vi "Main.vi"() -> ()   [LabVIEW 2018]
doc: "This Continuous Measurement sample project is based on the Queued Message Handler template.\n\nThe Event Handling Loop generates messages based on user interface actions.\n\nThe Message Handling Loop processes messages generated by the Event Handling Loop, or by other messages. There are also Acquisition and Logging message handling loop subVIs, and a chart updating loop."
uses:
  controls/UI Data.ctl
  controls/UI State.ctl
  support/Message Queue/Enqueue Message (Single).vi
  GlobalVariable/GlobalLongueurOnde.vi
  GlobalVariable/GlobalSet0.vi
  GlobalVariable/GlobalDefaultFolderPath.vi
  <vilib>/Utility/error.llb/Error Cluster From Error Code.vi
  <vilib>/ErrorRing/Error Ring.xnode
  Acquisition/Acquisition.lvlib
  support/User Event - Stop/User Event - Stop.lvlib
  support/Message Queue/Message Queue.lvlib
panel:
  out "Pos Y":dbl
  out "Pos X":dbl
  out "?":dbl[][](graph)
  in  "Mise à 0":bool
  in  "Longueur d'onde du laser":dbl
  in  "Exit":bool
  out "Data":waveform(dbl)[](graph)
  out "Array":variant[](array[variant])
  out "Status":string
  out "Puissance Instantannée":dbl
  in  "Start":bool
  in  "Stop":bool
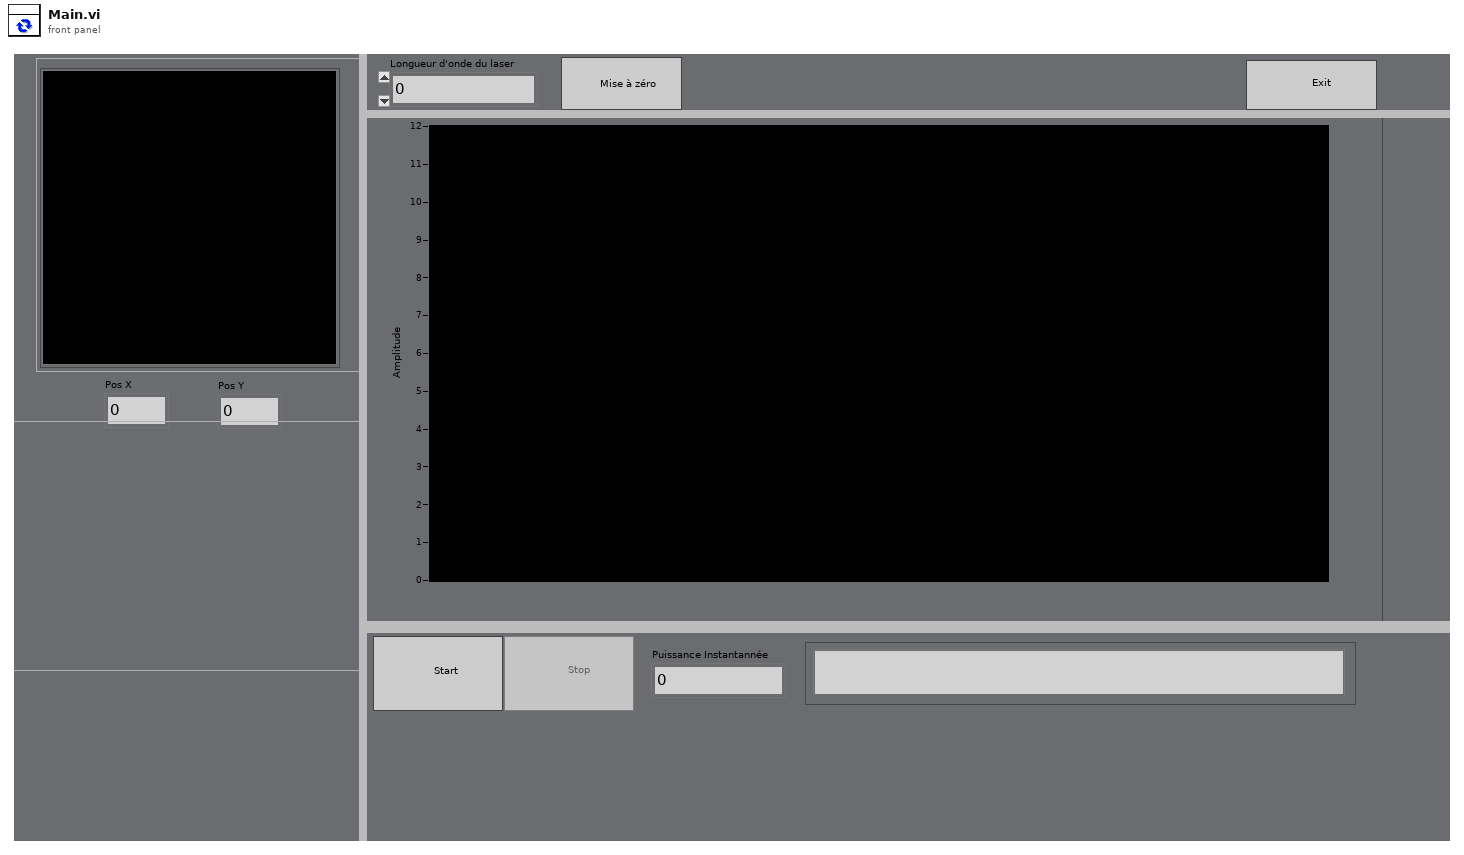
[diagram p1: front panel]
types:
  T1 = typedef "UI State.ctl" = enum16{"Idle", "Acquiring and Logging", "Waiting for Exit", "Waiting for Exit (Acq Stopped)", "Waiting for Exit (Log Stopped)", "Waiting for Stop", "Waiting for Stop (Acq Stopped)", "Waiting for Stop (Log Stopped)"}
  T2 = typedef "UI Data.ctl" = cluster{"Start Ref":refnum<vi>, "Stop Ref":refnum<vi>, "Settings Ref":refnum<vi>, "Exit Ref":refnum<vi>, "Status Ref":refnum<vi>, "Data Ref":refnum<vi>, "Longueur d'onde du laser":refnum<vi>, "Set 0 Ref":refnum<vi>}
  T3 = cluster{"UI":refnum<queue>, "Acquisition":refnum<queue>}
  T4 = enum16{"open", "replace", "create", "open or create", "replace or create", "replace or create with confirmation"}
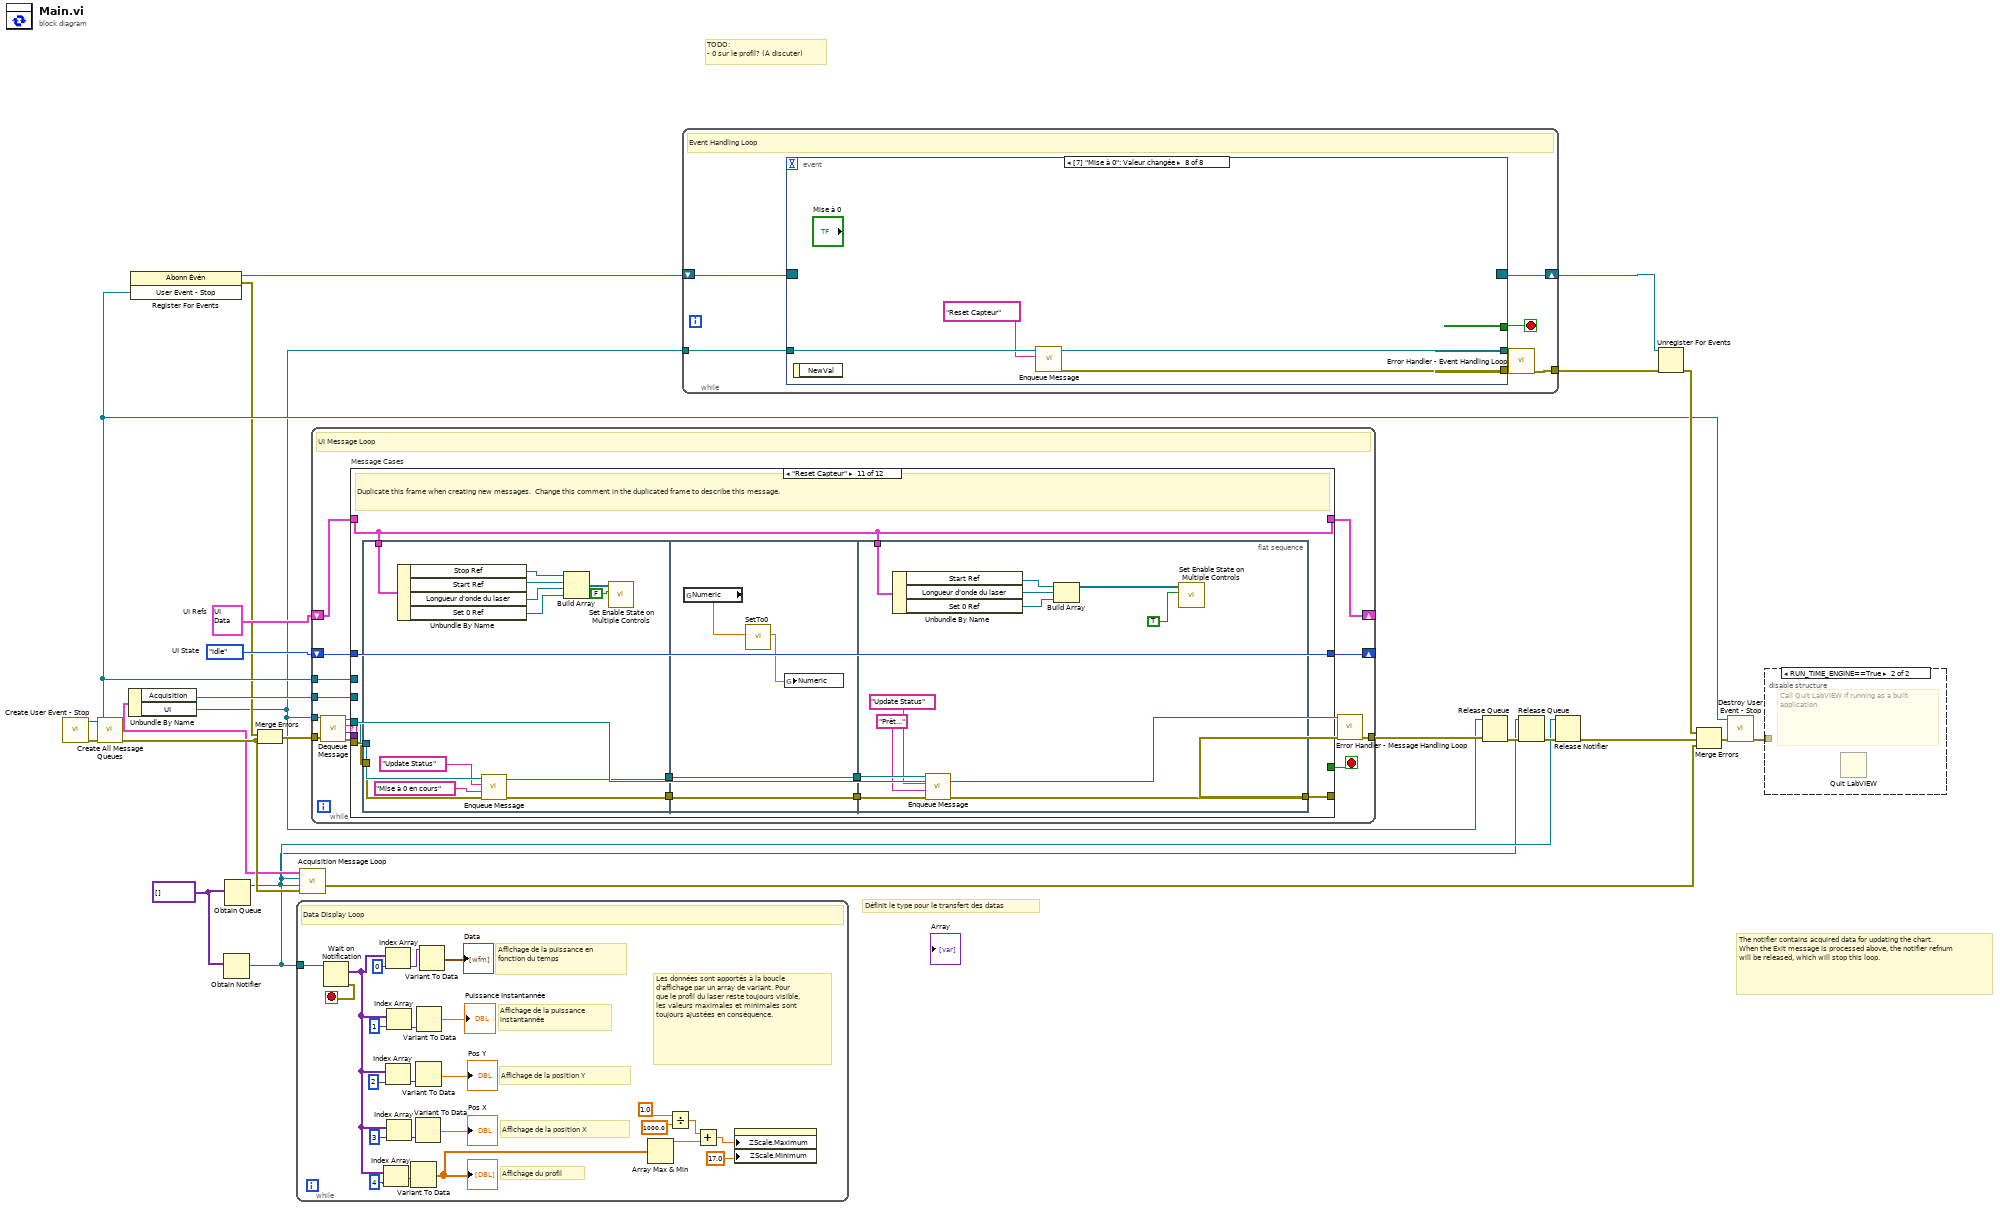
[diagram p0: block diagram]
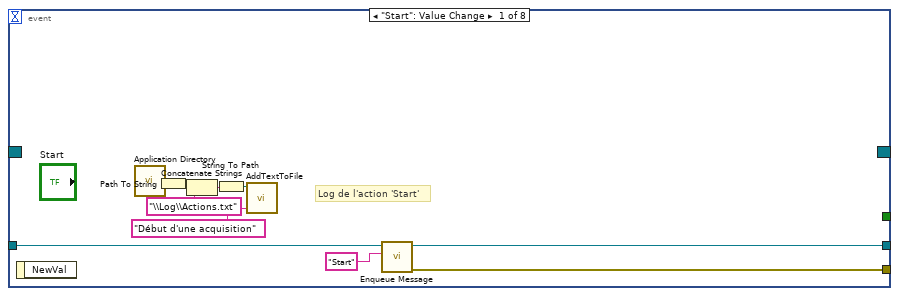
[diagram p3: hidden frame]
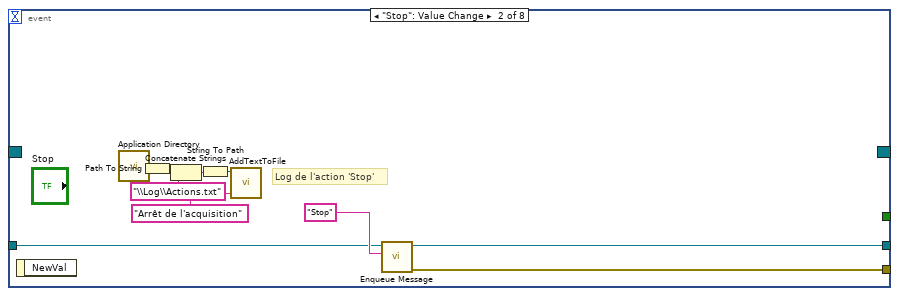
[diagram p4: hidden frame]
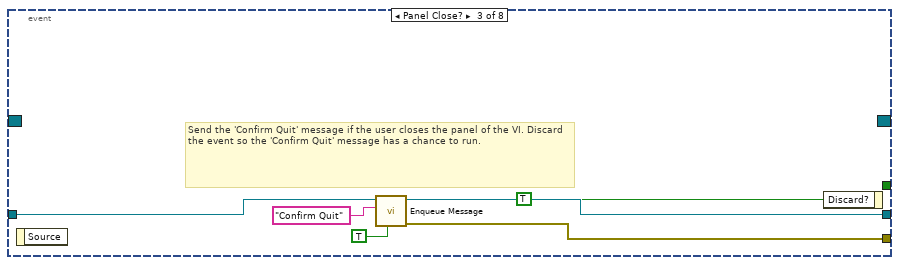
[diagram p5: hidden frame]
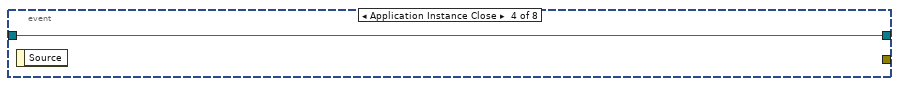
[diagram p6: hidden frame]
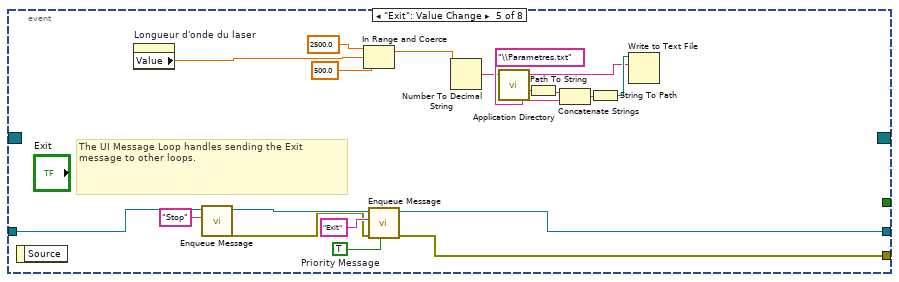
[diagram p7: hidden frame]
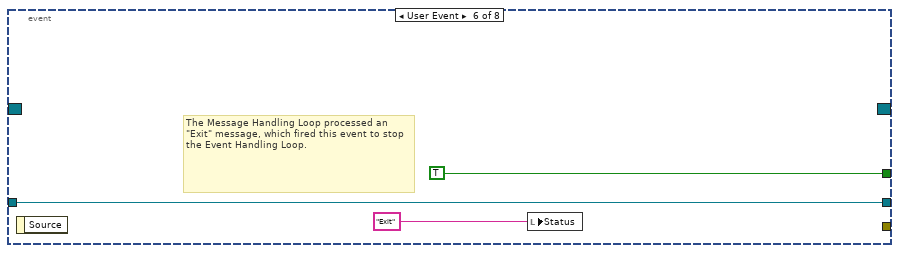
[diagram p8: hidden frame]
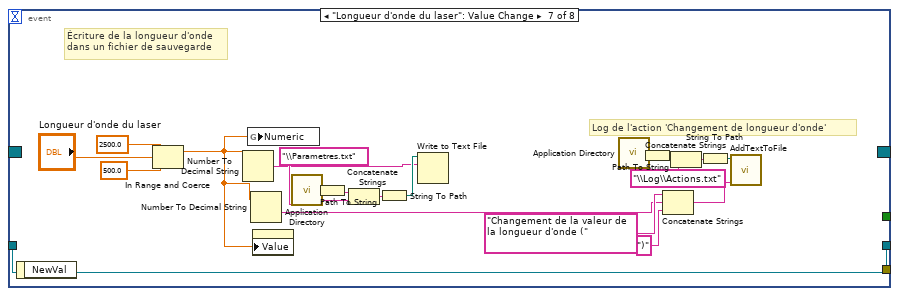
[diagram p9: hidden frame]
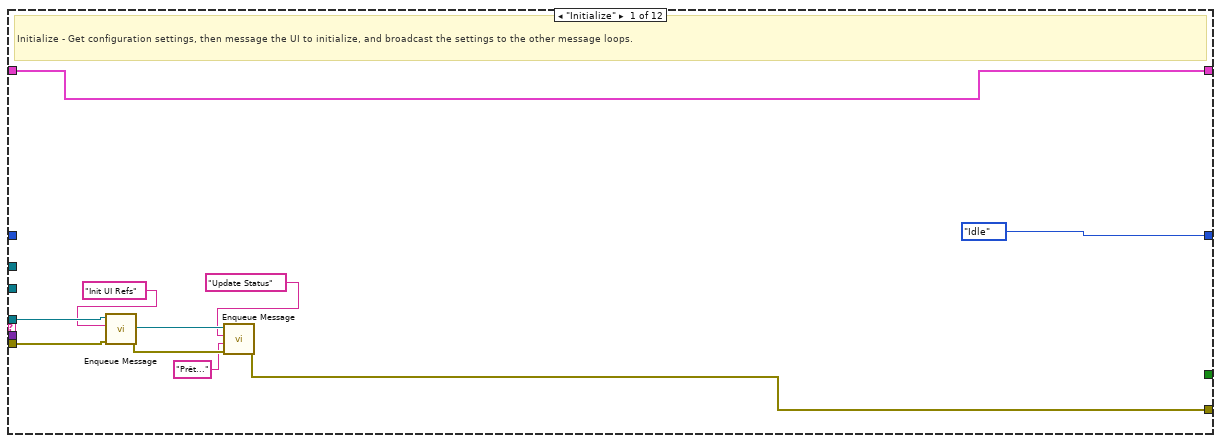
[diagram p10: hidden frame]
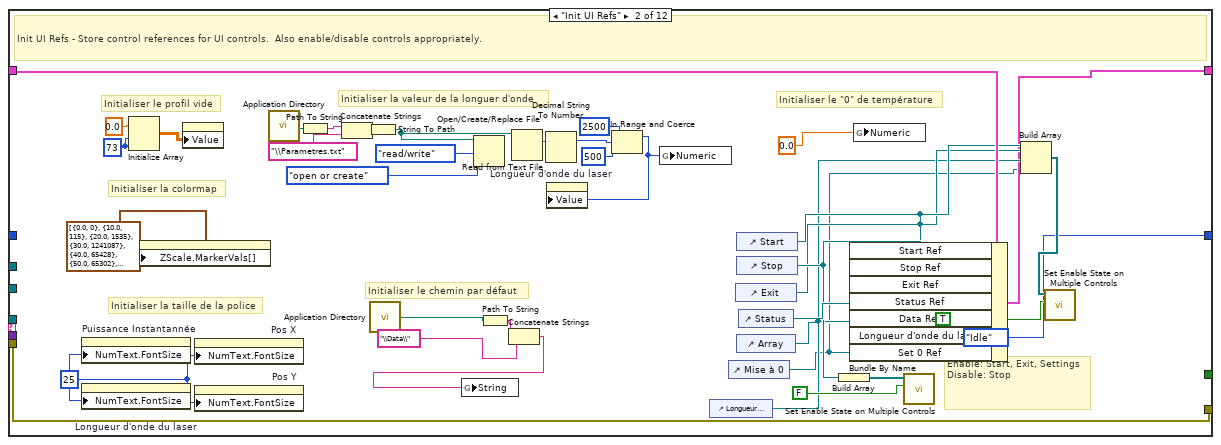
[diagram p11: hidden frame]
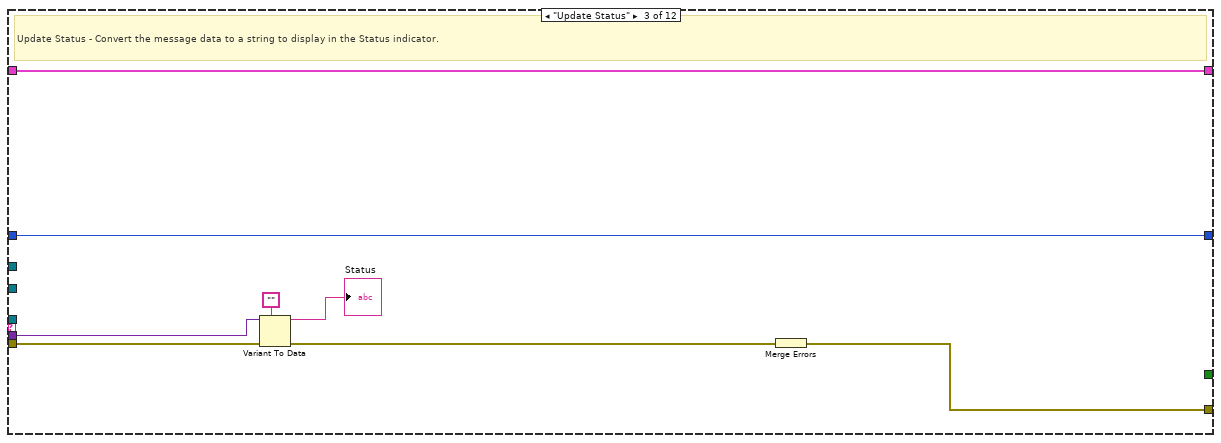
[diagram p12: hidden frame]
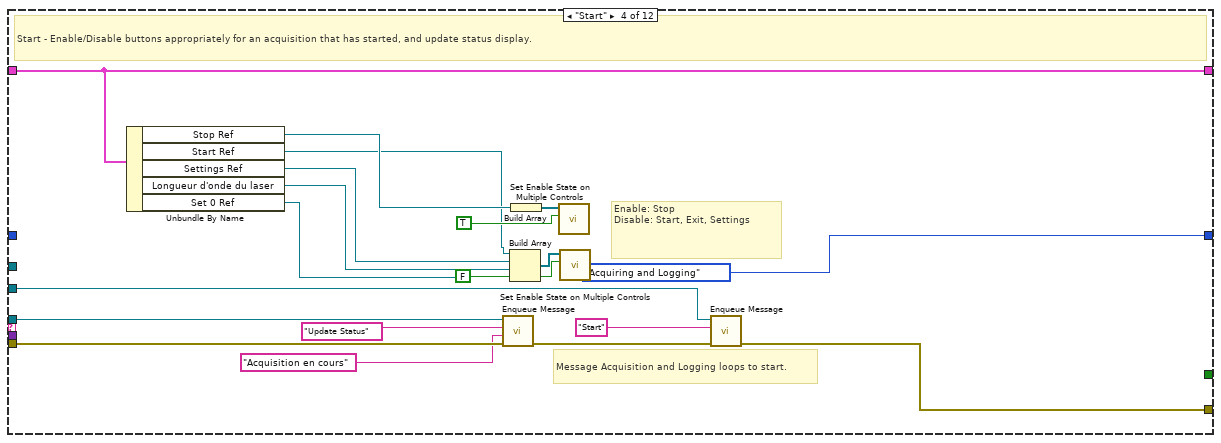
[diagram p13: hidden frame]
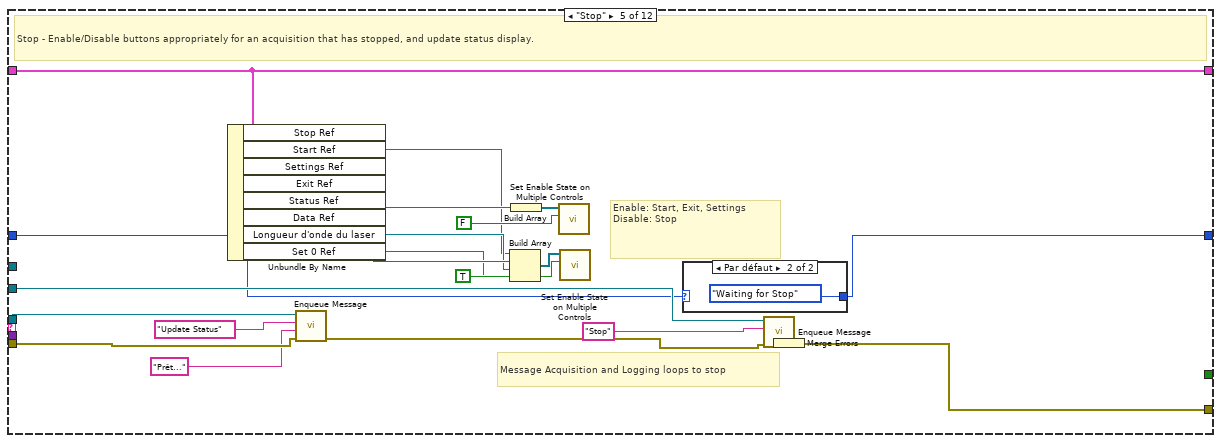
[diagram p14: hidden frame]
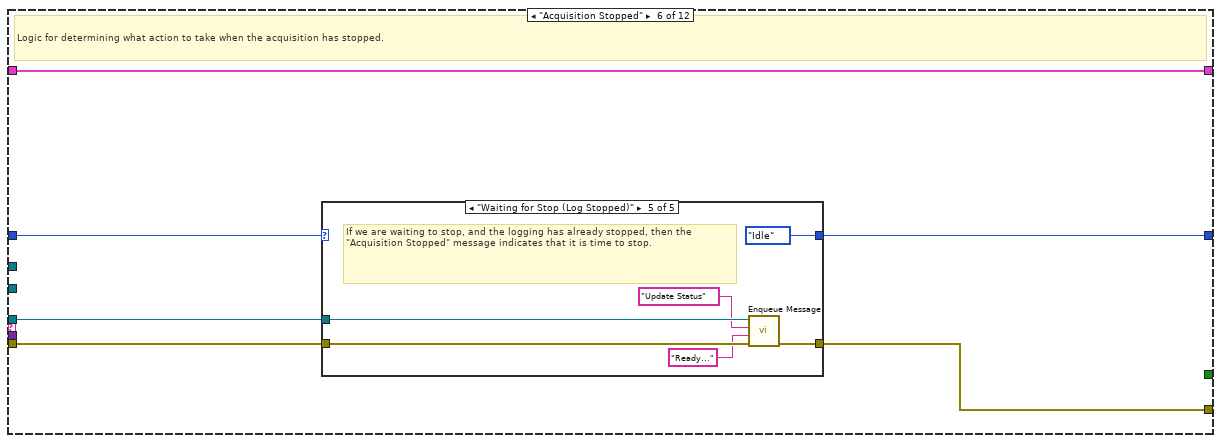
[diagram p16: hidden frame]
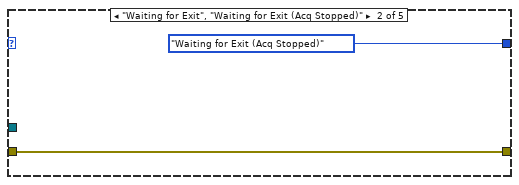
[diagram p18: hidden frame]
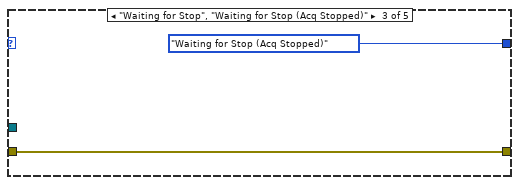
[diagram p19: hidden frame]
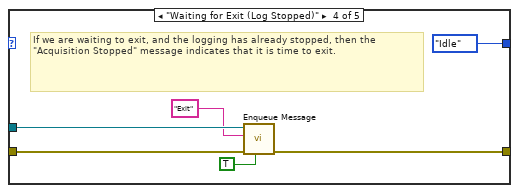
[diagram p20: hidden frame]
diagram:
  w3 = variant[] [] ("appended array")
  w16 = UI_State."Idle"  # UI State
  w18 = T2 {"Start Ref"=refnum, "Stop Ref"=refnum, "Settings Ref"=refnum, "Exit Ref"=refnum, "Status Ref"=refnum, "Data Ref"=refnum, "Longueur d'onde du laser"=refnum, "Set 0 Ref"=refnum}  # UI Refs
  # "TODO: \n- 0 sur le profil? (À discuter)"
  # "Définit le type pour le transfert des datas"
  # "The notifier contains acquired data for updating the chart. When the Exit message is processed above, the notifier refnum will be released, which will stop this loop."
  n1 = call "Create User Event - Stop.vi"() -> ("error out"=w21:errorcluster, "User Event - Stop"=w9:refnum<user-event>)  [unwired: 10 in]
  n2 = call "Create All Message Queues.vi"("error in (no error)"=w21) -> ("error out"=w20:errorcluster, "Message Queues out"=w4:T3)  [unwired: 9 in]
  n3 = Unbundle By Name(w4) -> ("Acquisition"=w17:refnum<queue>, "UI"=w6:refnum<queue>)
  n4 = register-events(w9) -> (reference out=w10:refnum<event-registration>, error out=w7:errorcluster)  [unwired: 2 in]
  n5 = Obtain Notifier(notification data type=w3) -> (notifier out=w2:refnum<notifier>)  [unwired: 3 in, 2 out]
  n6 = Obtain Queue(element data type=w3) -> (queue out=w1:refnum<queue>)  [unwired: 4 in, 2 out]
  n7 = Merge Errors(w7, w20) -> (w8:errorcluster)
  n8 = while "Data Display Loop" {
    tunnel: w2 -> [w48]
    stop <- w47 stop-if-true
    # "Les données sont apportés à la boucle d'affichage par un array de variant. Pour que le profil du laser reste toujours visible, les valeurs maximales et minimales sont toujours ajustées en conséquence."
    # "Affichage de la puissance en fonction du temps"
    # "Affichage de la position X"
    # "Affichage de la position Y"
    # "Affichage de la puissance\ninstantannée"
    # "Affichage du profil"
    # "Data Display Loop"
    n9 = Wait on Notification(notifier=w48) -> (notification=w36:variant[], error out=w47:errorcluster)  [unwired: 3 in, 2 out]
    n10 = Index Array(array=w36, index=4) -> (element=w34:variant)
    n11 = Index Array(array=w36, index=0) -> (element=w45:variant)
    n12 = Index Array(array=w36, index=2) -> (element=w40:variant)
    n13 = Index Array(array=w36, index=1) -> (element=w42:variant)
    n14 = Index Array(array=w36, index=3) -> (element=w37:variant)
    n15 = Variant To Data(Variant=w34) -> (data=w25:dbl[][])  [unwired: 2 in, 1 out]
    "?" <- w25
    n16 = Variant To Data(Variant=w37) -> (data=→"Pos X":dbl)  [unwired: 2 in, 1 out]
    n17 = Variant To Data(Variant=w40) -> (data=→"Pos Y":dbl)  [unwired: 2 in, 1 out]
    n18 = Variant To Data(Variant=w42) -> (data=→"Puissance Instantannée":dbl)  [unwired: 2 in, 1 out]
    n19 = Variant To Data(Variant=w45) -> (data=→"Data":waveform(dbl)[])  [unwired: 2 in, 1 out]
    n20 = Array Max & Min(array=w25) -> (max value=w33:dbl)  [unwired: 3 out]
    n21 = Divide(x=1.0, y=1000.0) -> (x/y=w32:dbl)
    n22 = Add(x=w32, y=w33) -> (x+y=w27:dbl)
    n23 = property class="GraphInt (strict)"("ZScale.Maximum"=w27, "ZScale.Minimum"=17.0 ("Z Scale.Range:Minimum")) -> ()  [unwired: 2 in, 2 out]
  }
  n24 = call "Acquisition Message Loop.vi"("error in (no error)"=w20, "queue out"=w1, "Data Notifier"=w2, "Message Queues"=w4) -> ("error out"=w22:errorcluster)  [unwired: 7 in]
  n25 = while {
    tunnel: w6 -> [w57]
    tunnel: w9 -> [w62]
    shift-right: [w55] -> _
    shift-left: w18 -> [w56]
    tunnel: w17 -> [w54]
    shift-right: [w49] -> _
    shift-left: w16 -> [w50]
    tunnel: w8 -> [w61]
    tunnel: [w53] -> w24
    stop <- w63 stop-if-true
    # "UI Message Loop"
    n26 = call "Dequeue Message.vi"("error in (no error)"=w61, "Message Queue"=w57) -> ("error out"=w60:errorcluster, "Message Data"=w58:variant, "Message"=w59:string, "dup Message Queue"=w51:refnum<queue>)  [unwired: 6 in]
    n27 = case "Message Cases" shown="\"Reset Capteur\"" w59 {
      selector: w59 -> [_ _ _ _ _ _ _ _ _ _ _ w274]
      tunnel: w51 -> [w68 _ _ w137 w143 w163 _ w196 _ _ w243 _]
      tunnel: w60 -> [w67 w110 w117 w136 w141 w164 w185 w195 _ w235 w242 _]
      tunnel: [w65 w110 w118 w126 w158 w161 w188 w194 w229 w234 w237 w273] -> w52
      tunnel: [_ _ _ _ _ _ _ _ TRUE _ _ _] -> w63
      tunnel: w58 -> [_ _ w116 _ _ _ w189 _ w224 _ _ _]
      tunnel: w62 -> [_ _ _ _ _ _ _ _ w230 _ _ _]
      tunnel: w56 -> [w69 w109 w112 w133 w157 w166 w192 w198 w228 w233 w236 w276]
      tunnel: [w69 w96 w112 w133 w157 w166 w192 w198 w228 w233 w236 w276] -> w55
      tunnel: w54 -> [_ _ _ w125 w149 _ _ _ w221 _ _ _]
      tunnel: w50 -> [_ _ w111 _ w146 w165 w187 w197 _ w232 w244 w275]
      tunnel: [UI_State."Idle" ("UI State") UI_State."Idle" ("UI State") w111 UI_State."Acquiring and Logging" ("UI State") w147 w162 w187 w193 UI_State."Idle" ("UI State") w232 w244 w275] -> w49
      frame "Initialize" {
        # "Initialize - Get configuration settings, then message the UI to initialize, and broadcast the settings to the other message loops."
        n28 = call-poly "Enqueue Message.vi"("error in (no error)"=w67, "Message"="Init UI Refs", "Message Queue"=w68) -> ("error out"=w73:errorcluster, "dup Message Queue"=w72:refnum<queue>)  [unwired: 7 in]
        n29 = call-poly "Enqueue Message.vi"("error in (no error)"=w73, "Message Data"="Prêt..." ("Ready..."), "Message"="Update Status", "Message Queue"=w72) -> ("error out"=w65:errorcluster)  [unwired: 6 in, 1 out]
      }
      frame "Init UI Refs" {
        w85 = 73 ("dimension size")
        w98 = 25
        # "Initialiser le \"0\" de température"
        # "Initialiser le profil vide"
        # "Initialiser la valeur de la longuer d'onde"
        # "Initialiser le chemin par défaut"
        # "Initialiser la colormap"
        # "Initialiser la taille de la police"
        # "Enable: Start, Exit, Settings\nDisable: Stop"
        # "Init UI Refs - Store control references for UI controls.  Also enable/disable controls appropriately."
        n30 = property on="Puissance Instantannée" class="NumNb (strict)"("NumText.FontSize"=w98) -> ()  [unwired: 2 in, 2 out]
        n31 = property on="Longueur d'onde du laser" class="NumNb (strict)"("NumText.FontSize"=w98) -> ()  [unwired: 2 in, 2 out]
        n32 = Initialize Array(0.0 ("element"), w85, w85) -> (w84:dbl[][])
        n33 = property class="GraphInt (strict)"("ZScale.MarkerVals[]"=cluster{dbl, u32}[] [{0.0, 0}, {10.0, 115}, {20.0, 1535}, {30.0, 1241087}, {40.0, 65428}, {50.0, 65302}, {60.0, 15925010}, {70.0, 16756736}, {80.0, 16739858}, {90.0, 16712704}, {100.0, 10420224}] ("Z Scale.Marker Values[]")) -> ()  [unwired: 2 in, 2 out]
        n34 = property class="GraphInt (strict)"("Value"=w84) -> ()  [unwired: 2 in, 2 out]
        n35 = property on="Pos X" class="NumNb (strict)"("NumText.FontSize"=w98) -> ()  [unwired: 2 in, 2 out]
        n36 = property on="Pos Y" class="NumNb (strict)"("NumText.FontSize"=w98) -> ()  [unwired: 2 in, 2 out]
        n37 = call <vilib>:"Application Directory.vi"() -> ("Application Directory"=w92:path)
        n38 = Path To String(path=w92) -> (string=w91:string)
        n39 = Concatenate Strings(w91, "\\Parametres.txt") -> (w90:string)
        n40 = String To Path(string=w90) -> (path=w78:path)
        n41 = call <vilib>:"Application Directory.vi"() -> ("Application Directory"=w95:path)
        n42 = Open/Create/Replace File(file path (use dialog)=w78, operation (0:open)=T4."open or create", access (0:read/write)=enum16{"read/write", "read-only", "write-only"}."read/write") -> ()  [unwired: 3 in, 3 out]
        n43 = Path To String(path=w95) -> (string=w94:string)
        n44 = Concatenate Strings(w94, "\\Data\\") -> (w82:string)
        n45 = global write "GlobalDefaultFolderPath.vi" "String"(w82) -> ()
        n46 = Read from Text File(file (use dialog)=w78) -> (text=w88:string)  [unwired: 3 in, 3 out]
        n47 = Decimal String To Number(string=w88) -> (number=w81:i32)  [unwired: 2 in, 1 out]
        n48 = In Range and Coerce(upper limit=2500, x=w81, lower limit=500) -> (coerced(x)=w75:i32)  [unwired: 1 out]
        n49 = property on="Longueur d'onde du laser" class="NumNb (strict)"("Value"=w75) -> ()  [unwired: 2 in, 2 out]
        n50 = global write "GlobalLongueurOnde.vi" "Numeric"(w75) -> ()
        n51 = control-ref of="Longueur d'onde du laser"() -> (w99:refnum<vi>)
        n52 = control-ref of="Mise à 0"() -> (w83:refnum<vi>)
        n53 = control-ref of="Exit"() -> (w101:refnum<vi>)
        n54 = control-ref of="Start"() -> (w102:refnum<vi>)
        n55 = control-ref of="Stop"() -> (w103:refnum<vi>)
        n56 = control-ref of="Array"() -> (w87:refnum<vi>)
        n57 = control-ref of="Status"() -> (w108:refnum<vi>)
        n58 = Build Array(w103) -> (w105:refnum<vi>[])
        n59 = Bundle By Name(cluster=w109, "Start Ref"=w102, "Stop Ref"=w103, "Exit Ref"=w101, "Status Ref"=w108, "Data Ref"=w87, "Longueur d'onde du laser"=w99, "Set 0 Ref"=w83) -> (w96:T2)
        n60 = global write "GlobalSet0.vi" "Numeric"(0.0 ("Temp Ambiant")) -> ()
        n61 = call "Set Enable State on Multiple Controls.vi"("Enable?"=FALSE, "Controls"=w105) -> ()  [unwired: 10 in]
        n62 = Build Array(w102, w101, w99, w83) -> (w106:refnum<vi>[])
        n63 = call "Set Enable State on Multiple Controls.vi"("Enable?"=TRUE, "Controls"=w106) -> ()  [unwired: 10 in]
      }
      frame "Update Status" {
        # "Update Status - Convert the message data to a string to display in the Status indicator."
        n64 = Variant To Data(error in=w117, type="", Variant=w116) -> (data=→"Status":string, error out=w114:errorcluster)
        n65 = Merge Errors(w114) -> (w118:errorcluster)
      }
      frame "Start" {
        # "Message Acquisition and Logging loops to start."
        # "Enable: Stop\nDisable: Start, Exit, Settings"
        # "Start - Enable/Disable buttons appropriately for an acquisition that has started, and update status display."
        n66 = Unbundle By Name(w133) -> ("Stop Ref"=w128:refnum<vi>, "Start Ref"=w121:refnum<vi>, "Settings Ref"=w127:refnum<vi>, "Longueur d'onde du laser"=w122:refnum<vi>, "Set 0 Ref"=w119:refnum<vi>)
        n67 = call-poly "Enqueue Message.vi"("error in (no error)"=w136, "Message Data"="Acquisition en cours" ("Acquiring and Logging..."), "Message"="Update Status", "Message Queue"=w137) -> ("error out"=w120:errorcluster)  [unwired: 6 in, 1 out]
        n68 = Build Array(w121, w127, w122, w119) -> (w131:refnum<vi>[])
        n69 = Build Array(w128) -> (w130:refnum<vi>[])
        n70 = call "Set Enable State on Multiple Controls.vi"("Enable?"=TRUE, "Controls"=w130) -> ()  [unwired: 10 in]
        n71 = call "Set Enable State on Multiple Controls.vi"("Enable?"=FALSE, "Controls"=w131) -> ()  [unwired: 10 in]
        n72 = call-poly "Enqueue Message.vi"("error in (no error)"=w120, "Message"="Start", "Message Queue"=w125) -> ("error out"=w126:errorcluster)  [unwired: 7 in, 1 out]
      }
      frame "Stop" {
        # "Message Acquisition and Logging loops to stop"
        # "Enable: Start, Exit, Settings\nDisable: Stop"
        # "Stop - Enable/Disable buttons appropriately for an acquisition that has stopped, and update status display."
        n73 = Unbundle By Name(w157) -> ("Stop Ref"=w152:refnum<vi>, "Start Ref"=w144:refnum<vi>, "Settings Ref"=w151:refnum<vi>, "Longueur d'onde du laser"=w145:refnum<vi>, "Set 0 Ref"=w138:refnum<vi>)  [unwired: 3 out]
        n74 = call-poly "Enqueue Message.vi"("error in (no error)"=w141, "Message Data"="Prêt..." ("Acquiring and Logging..."), "Message"="Update Status", "Message Queue"=w143) -> ("error out"=w139:errorcluster)  [unwired: 6 in, 1 out]
        n75 = Build Array(w144, w151, w145, w138) -> (w155:refnum<vi>[])
        n76 = Build Array(w152) -> (w154:refnum<vi>[])
        n77 = call "Set Enable State on Multiple Controls.vi"("Enable?"=FALSE, "Controls"=w154) -> ()  [unwired: 10 in]
        n78 = call "Set Enable State on Multiple Controls.vi"("Enable?"=TRUE, "Controls"=w155) -> ()  [unwired: 10 in]
        n79 = case shown="Par défaut" w146 {
          selector: w146 -> [w159 _]
          tunnel: [w159 UI_State."Waiting for Stop" ("UI State")] -> w147
          frame "Waiting for Exit" {
          }
          frame Default {
          }
        }
        n80 = call-poly "Enqueue Message.vi"("error in (no error)"=w139, "Message"="Stop", "Message Queue"=w149) -> ("error out"=w150:errorcluster)  [unwired: 7 in, 1 out]
        n81 = Merge Errors(w150) -> (w158:errorcluster)
      }
      frame "Acquisition Stopped" {
        # "Logic for determining what action to take when the acquisition has stopped."
        n82 = case shown="\"Waiting for Stop (Log Stopped)\"" w165 {
          selector: w165 -> [w168 _ _ _ _]
          tunnel: w164 -> [w167 w170 w172 w178 w184]
          tunnel: w163 -> [_ _ _ w176 w181]
          tunnel: [w168 UI_State."Waiting for Exit (Acq Stopped)" ("UI State") UI_State."Waiting for Stop (Acq Stopped)" ("UI State") UI_State."Idle" ("UI State") UI_State."Idle" ("UI State")] -> w162
          tunnel: [w167 w170 w172 w177 w182] -> w161
          frame Default {
          }
          frame "Waiting for Exit", "Waiting for Exit (Acq Stopped)" {
          }
          frame "Waiting for Stop", "Waiting for Stop (Acq Stopped)" {
          }
          frame "Waiting for Exit (Log Stopped)" {
            # "If we are waiting to exit, and the logging has already stopped, then the \"Acquisition Stopped\" message indicates that it is time to exit."
            n83 = call-poly "Enqueue Message.vi"("Priority Message? (F)"=TRUE, "error in (no error)"=w178, "Message"="Exit", "Message Queue"=w176) -> ("error out"=w177:errorcluster)  [unwired: 6 in, 1 out]
          }
          frame "Waiting for Stop (Log Stopped)" {
            # "If we are waiting to stop, and the logging has already stopped, then the \"Acquisition Stopped\" message indicates that it is time to stop."
            n84 = call-poly "Enqueue Message.vi"("error in (no error)"=w184, "Message Data"="Ready..." ("Ready..."), "Message"="Update Status", "Message Queue"=w181) -> ("error out"=w182:errorcluster)  [unwired: 6 in, 1 out]
          }
        }
      }
      frame "Error" {
        # "Error - Display an error dialog. This message is sent by the \"Error Handler\" VIs at the end of other loops in this application."
        n85 = Variant To Data(error in=w185, type=errorcluster {"status"=FALSE, "code"=0, "source"=""} ("error constant"), Variant=w189) -> (data=w186:errorcluster, error out=w190:errorcluster)
        n86 = call <vilib>:"Simple Error Handler.vi"("error in (no error)"=w186) -> ()  [unwired: 4 in, 5 out]
        n87 = Merge Errors(w190) -> (w188:errorcluster)
      }
      frame "Confirm Quit" {
        # "Confirm Quit - Message that can confirm whether or not the user wants to exit the application."
        n88 = case shown="\"Acquiring and Logging\"" w197 {
          tunnel: w196 -> [w204 w208]
          tunnel: w195 -> [w203 w207]
          tunnel: [w202 w206] -> w194
          tunnel: [UI_State."Idle" ("UI State") w205] -> w193
          frame Default {
            # "If 'Confirm Quit' comes in while the system is idle, there is no need for a confirmation message."
            n89 = call-poly "Enqueue Message.vi"("Priority Message? (F)"=TRUE, "error in (no error)"=w203, "Message"="Exit", "Message Queue"=w204) -> ("error out"=w202:errorcluster)  [unwired: 6 in, 1 out]
          }
          frame "Acquiring and Logging" {
            n90 = Two Button Dialog(message="Are you sure you want to quit while the acquisition is running?" ("Confirm Quit Message"), 1:"No" ("No"), 2:"Yes" ("Yes")) -> (T button?=w209:bool)
            n91 = case shown="Vrai" w209 {
              tunnel: w208 -> [_ w218]
              tunnel: w207 -> [w214 w219]
              tunnel: [w214 w217] -> w206
              tunnel: [UI_State."Acquiring and Logging" ("UI State") UI_State."Waiting for Exit" ("UI State")] -> w205
              frame False {
                # "User did not want to quit."
              }
              frame True {
                n92 = call-poly "Enqueue Message.vi"("error in (no error)"=w219, "Message"="Stop", "Message Queue"=w218) -> ("error out"=w217:errorcluster)  [unwired: 7 in, 1 out]
              }
            }
          }
        }
      }
      frame "Exit" {
        # "Popup an error dialog if 'Exit' was called as a result of an error."
        # "Stop the VI"
        # "Exit - Send Exit messages to the Acquisition and Logging loops, and fire the user event to stop the Event Handling Loop."
        n93 = Variant To Data(type=errorcluster {"status"=FALSE, "code"=0, "source"=""} ("error constant"), Variant=w224) -> (data=w223:errorcluster)  [unwired: 1 in, 1 out]
        n94 = call <vilib>:"Simple Error Handler.vi"("error in (no error)"=w223) -> ()  [unwired: 4 in, 5 out]
        n95 = call-poly "Enqueue Message.vi"("Priority Message? (F)"=FALSE, "Message"="Exit", "Message Queue"=w221) -> ("error out"=w220:errorcluster)  [unwired: 7 in, 1 out]
        n96 = call "Fire User Event - Stop.vi"("error in (no error)"=w220, "User Event - Stop"=w230) -> ("error out"=w229:errorcluster)  [unwired: 9 in]
      }
      frame "---Copy This Frame---" {
        # "Duplicate this frame when creating new messages.  Change this comment in the duplicated frame to describe this message."
        n97 = Merge Errors(w235) -> (w234:errorcluster)
      }
      frame "Reset Capteur" {
        # "Duplicate this frame when creating new messages.  Change this comment in the duplicated frame to describe this message."
        n98 = flat-sequence {
          tunnel: w243 -> [w257]
          tunnel: w242 -> [w256]
          tunnel: [w253] -> w241
          tunnel: [w252] -> w238
          tunnel: w236 -> [w251]
          tunnel: w241 -> [w259]
          tunnel: [w259] -> w240
          tunnel: [w258] -> w239
          tunnel: w238 -> [w258]
          tunnel: w240 -> [w272]
          tunnel: w239 -> [w271]
          tunnel: [w268] -> w237
          tunnel: w236 -> [w267]
          frame #0 {
            n99 = Unbundle By Name(w251) -> ("Stop Ref"=w250:refnum<vi>, "Start Ref"=w249:refnum<vi>, "Longueur d'onde du laser"=w248:refnum<vi>, "Set 0 Ref"=w247:refnum<vi>)
            n100 = call-poly "Enqueue Message.vi"("error in (no error)"=w256, "Message Data"="Mise à 0 en cours" ("Message"), "Message"="Update Status", "Message Queue"=w257) -> ("error out"=w252:errorcluster, "dup Message Queue"=w253:refnum<queue>)  [unwired: 6 in]
            n101 = Build Array(w250, w249, w248, w247) -> (w246:refnum<vi>[])
            n102 = call "Set Enable State on Multiple Controls.vi"("Enable?"=FALSE, "Controls"=w246) -> ()  [unwired: 10 in]
          }
          frame #1 {
            n103 = global read "GlobalLongueurOnde.vi" "Numeric"() -> (w261:dbl)
            n104 = call "SetTo0.vi"("Longueur d'onde"=w261) -> ("Température 0"=w260:dbl)  [unwired: 10 in]
            n105 = global write "GlobalSet0.vi" "Numeric"(w260) -> ()
          }
          frame #2 {
            n106 = Unbundle By Name(w267) -> ("Start Ref"=w266:refnum<vi>, "Longueur d'onde du laser"=w265:refnum<vi>, "Set 0 Ref"=w264:refnum<vi>)
            n107 = call-poly "Enqueue Message.vi"("error in (no error)"=w271, "Message Data"="Prêt..." ("Message"), "Message"="Update Status", "Message Queue"=w272) -> ("error out"=w268:errorcluster)  [unwired: 6 in, 1 out]
            n108 = Build Array(w266, w265, w264) -> (w263:refnum<vi>[])
            n109 = call "Set Enable State on Multiple Controls.vi"("Enable?"=TRUE, "Controls"=w263) -> ()  [unwired: 10 in]
          }
        }
      }
      frame Default {
        # "'Default' case only runs if there is a message that isn't defined in any of the other cases.  Output a programming error."
        n110 = xnode "Error Ring"("paramètre 0"=w274) -> ("sortie d'erreur"=w273:errorcluster)
      }
    }
    n111 = call "Error Handler - Message Handling Loop.vi"("error in (no error)"=w52, "Message Queue"=w51) -> ("dup error in"=w53:errorcluster)  [unwired: 8 in, 1 out]
  }
  n112 = while {
    tunnel: w6 -> [w289]
    tunnel: [w286] -> w23
    shift-right: [w288] -> w5
    shift-left: w10 -> [w290]
    stop <- w287 stop-if-true
    # "Event Handling Loop"
    n113 = event shown="[7] \"Mise à 0\": Valeur changée" {
      selector: w290 -> [_ _ _ _ _ _ _ _]
      dyn-events: [_ _ _ _ _ _ _ _] -> w288
      timeout: _ -> [_ _ _ _ _ _ _ _]
      tunnel: [_ _ _ _ _ TRUE ("Discard?") _ _] -> w287
      tunnel: w289 -> [w300 w309 w314 w317 w331 w336 w358 w362]
      tunnel: [w298 w308 w312 _ w335 _ _ w360] -> w285
      tunnel: [w297 w307 w313 w317 w332 w336 w358 w361] -> w284
      event "Start": Value Change {
        # "Log de l'action 'Start'"
        n114 = event-data() -> ()  [unwired: 1 in, 1 out]
        n115 = call <vilib>:"Application Directory.vi"() -> ("Application Directory"=w294:path)
        n116 = Path To String(path=w294) -> (string=w295:string)
        n117 = Concatenate Strings(w295, "\\Log\\Actions.txt") -> (w296:string)
        n118 = String To Path(string=w296) -> (path=w292:path)
        n119 = call "AddTextToFile.vi"("Ajouter du texte"="Début d'une acquisition", "Fichier"=w292) -> ()  [unwired: 10 in]
        n120 = call-poly "Enqueue Message.vi"("Message"="Start", "Message Queue"=w300) -> ("error out"=w298:errorcluster, "dup Message Queue"=w297:refnum<queue>)  [unwired: 8 in]
      }
      event "Stop": Value Change {
        # "Log de l'action 'Stop'"
        n121 = event-data() -> ()  [unwired: 1 in, 1 out]
        n122 = call <vilib>:"Application Directory.vi"() -> ("Application Directory"=w304:path)
        n123 = Path To String(path=w304) -> (string=w305:string)
        n124 = Concatenate Strings(w305, "\\Log\\Actions.txt") -> (w306:string)
        n125 = String To Path(string=w306) -> (path=w302:path)
        n126 = call "AddTextToFile.vi"("Ajouter du texte"="Arrêt de l'acquisition", "Fichier"=w302) -> ()  [unwired: 10 in]
        n127 = call-poly "Enqueue Message.vi"("Message"="Stop", "Message Queue"=w309) -> ("error out"=w308:errorcluster, "dup Message Queue"=w307:refnum<queue>)  [unwired: 8 in]
      }
      event Panel Close? {
        # "Send the 'Confirm Quit' message if the user closes the panel of the VI. Discard the event so the 'Confirm Quit' message has a chance to run."
        n128 = event-data() -> ()  [unwired: 1 in, 1 out]
        n129 = call-poly "Enqueue Message.vi"("Priority Message? (F)"=TRUE, "Message"="Confirm Quit", "Message Queue"=w314) -> ("error out"=w312:errorcluster, "dup Message Queue"=w313:refnum<queue>)  [unwired: 7 in]
        n130 = event-data("Discard?"=TRUE) -> ()  [unwired: 1 in, 1 out]
      }
      event Application Instance Close {
        n131 = event-data() -> ()  [unwired: 1 in, 1 out]
      }
      event "Exit": Value Change {
        w333 = TRUE  # Priority Message
        # "The UI Message Loop handles sending the Exit message to other loops."
        n132 = event-data() -> ()  [unwired: 1 in, 1 out]
        n133 = property on="Longueur d'onde du laser" class="NumNb (strict)"() -> ("Value"=w318:dbl)  [unwired: 2 in, 2 out]
        n134 = call-poly "Enqueue Message.vi"("Message"="Stop", "Message Queue"=w331) -> ("error out"=w329:errorcluster, "dup Message Queue"=w330:refnum<queue>)  [unwired: 8 in]
        n135 = In Range and Coerce(upper limit=2500.0, x=w318, lower limit=500.0) -> (coerced(x)=w320:dbl)  [unwired: 1 out]
        n136 = call-poly "Enqueue Message.vi"("Priority Message? (F)"=w333, "error in (no error)"=w329, "Message"="Exit", "Message Queue"=w330) -> ("error out"=w335:errorcluster, "dup Message Queue"=w332:refnum<queue>)  [unwired: 6 in]
        n137 = Number To Decimal String(number=w320) -> (decimal integer string=w322:string)  [unwired: 1 in]
        n138 = call <vilib>:"Application Directory.vi"() -> ("Application Directory"=w327:path)
        n139 = Path To String(path=w327) -> (string=w326:string)
        n140 = Concatenate Strings(w326, "\\Parametres.txt") -> (w324:string)
        n141 = String To Path(string=w324) -> (path=w323:path)
        n142 = Write to Text File(file (use dialog)=w323, text=w322) -> ()  [unwired: 2 in, 3 out]
      }
      event User Event {
        # "The Message Handling Loop processed an \"Exit\" message, which fired this event to stop the Event Handling Loop."
        n143 = event-data() -> ()  [unwired: 1 in, 1 out]
        n144 = local write "Status"("Exit" ("Exit String")) -> ()
      }
      event "Longueur d'onde du laser": Value Change {
        # "Log de l'action 'Changement de longueur d'onde'"
        # "Écriture de la longueur d'onde\ndans un fichier de sauvegarde"
        n145 = event-data() -> ()  [unwired: 1 in, 1 out]
        n146 = In Range and Coerce(upper limit=2500.0, x="Longueur d'onde du laser", lower limit=500.0) -> (coerced(x)=w339:dbl)  [unwired: 1 out]
        n147 = Number To Decimal String(number=w339) -> (decimal integer string=w352:string)  [unwired: 1 in]
        n148 = global write "GlobalLongueurOnde.vi" "Numeric"(w339) -> ()
        n149 = Number To Decimal String(number=w339) -> (decimal integer string=w345:string)  [unwired: 1 in]
        n150 = property on="Longueur d'onde du laser" class="NumNb (strict)"("Value"=w339) -> ()  [unwired: 2 in, 2 out]
        n151 = call <vilib>:"Application Directory.vi"() -> ("Application Directory"=w357:path)
        n152 = Path To String(path=w357) -> (string=w356:string)
        n153 = Concatenate Strings(w356, "\\Parametres.txt") -> (w354:string)
        n154 = String To Path(string=w354) -> (path=w353:path)
        n155 = Write to Text File(file (use dialog)=w353, text=w352) -> ()  [unwired: 2 in, 3 out]
        n156 = call <vilib>:"Application Directory.vi"() -> ("Application Directory"=w349:path)
        n157 = Path To String(path=w349) -> (string=w350:string)
        n158 = Concatenate Strings("Changement de la valeur de la longueur d'onde (" ("Ajouter du texte"), w345, ")" ("string")) -> (w343:string)
        n159 = Concatenate Strings(w350, "\\Log\\Actions.txt") -> (w351:string)
        n160 = String To Path(string=w351) -> (path=w347:path)
        n161 = call "AddTextToFile.vi"("Ajouter du texte"=w343, "Fichier"=w347) -> ()  [unwired: 10 in]
      }
      event "Mise à 0": Value Change {
        n162 = event-data() -> ()  [unwired: 1 in, 1 out]
        n163 = call-poly "Enqueue Message.vi"("Message"="Reset Capteur", "Message Queue"=w362) -> ("error out"=w360:errorcluster, "dup Message Queue"=w361:refnum<queue>)  [unwired: 8 in]
      }
    }
    n164 = call "Error Handler - Event Handling Loop.vi"("error in (no error)"=w285, "Message Queue"=w284) -> ("dup error in"=w286:errorcluster)  [unwired: 8 in, 1 out]
  }
  n165 = Release Queue(queue=w6, error in (no error)=w24) -> (error out=w13:errorcluster)  [unwired: 1 in, 2 out]
  n166 = Release Queue(queue=w1, error in (no error)=w13) -> (error out=w12:errorcluster)  [unwired: 1 in, 2 out]
  n167 = Release Notifier(notifier=w2, error in (no error)=w12) -> (error out=w11:errorcluster)  [unwired: 1 in, 2 out]
  n168 = Unregister For Events(event registration refnum=w5, error in=w23) -> (error out=w19:errorcluster)
  n169 = Merge Errors(w19, w11, w22) -> (w15:errorcluster)
  n170 = call "Destroy User Event - Stop.vi"("error in (no error)"=w15, "User Event - Stop"=w9) -> ("error out"=w14:errorcluster)  [unwired: 9 in]
  n171 = disable-structure shown="RUN_TIME_ENGINE==True" {
    disable-tunnel: w14 -> [_ _]
    frame condition #0 (active) {
    }
    frame condition #1 {
      # "Call Quit LabVIEW if running as a built application."
      n172 = Quit LabVIEW() -> ()  [unwired: 1 in]
    }
  }
